vi "Main.vi"(11 "Module Admin":refnum<class "Delacor_lib_QMH_Cloneable Module Admin.lvclass">) -> ()   [LabVIEW 2024, in "CTIWrapper.lvlib"]
doc: "This template is based off of the Queued Message Handler design pattern and the Queued Message Handler project template that ships with LabVIEW.\n\nThe main difference is that the queue is private to this module and communication between modules is performed via Broadcast and Request events.\n\nRequest events are wrapped in public API methods and are handled in the Event Handling Loop (EHL) of this VI. Any module can register for Broadcast events sent by this module. The EHL generates messages based on user interface actions.\n\nThe Message Handling Loop (MHL) processes messages generated by the EHL, or by other messages. The messages are string values, so new messages can be added easily to the Message Cases case structure in the MHL. Each message cluster can also provide an optional value for Message Data, which is a variant that can be converted to whatever message-specific data is required.\n_____\nBased on DQMH Dev Tools: Project Template 7.1.0.1503."
uses:
  CTIWrapper.lvlib
  <vilib>/Delacor/Delacor QMH/Libraries/Cloneable Module Admin_class/Delacor_lib_QMH_Cloneable Module Admin.lvclass
  C:/Program Files (x86)/National Instruments/LabVIEW 2024/vi.lib/Delacor/Delacor QMH/Libraries/Module Admin_class/Delacor_lib_QMH_Module Admin.lvclass
  Module Data--cluster.ctl
  <vilib>/Delacor/Delacor QMH/Libraries/Cloneable Module Admin_class/Delacor_lib_QMH_Cloneable Module Admin.lvclass/Delacor_lib_QMH_Cloneable Module Admin.ctl
  <vilib>/Delacor/Delacor QMH/Libraries/Message Queue_class/Delacor_lib_QMH_Message Queue.lvclass/Delacor_lib_QMH_Message Queue.ctl
  Stop Argument--cluster.ctl
  <vilib>/Delacor/Delacor QMH/Libraries/Module Admin_class/Delacor_lib_QMH_Module Admin.lvclass/Delacor_lib_QMH_Module Admin.ctl
  Initialize Device Argument--cluster.ctl
  Initialize Device (Reply Payload)--cluster.ctl
  <instrlib>/HandsOnPi2040/cti-drivers-lv-visa-main/CTI-Visa/Identity.ctl
  Set DO Argument--cluster.ctl
  Close Device Argument--cluster.ctl
  <vilib>/Utility/miscctls.llb/LVPointTypeDef.ctl
  <vilib>/Delacor/Delacor QMH/Libraries/Message Queue_class/Delacor_lib_QMH_Enqueue Message (Single).vi
  <vilib>/Delacor/Delacor QMH/Libraries/Cloneable Module Admin_class/Delacor_lib_QMH_Get Module ID.vi
  <vilib>/Delacor/Delacor QMH/Libraries/Module Admin_class/Delacor_lib_QMH_Get External Launch.vi
  <vilib>/Delacor/Delacor QMH/Libraries/Message Queue_class/Delacor_lib_QMH_Message Queue.lvclass
  <instrlib>/HandsOnPi2040/cti-drivers-lv-visa-main/CTI-Visa/CTI-Visa.lvlib
  <instrlib>/HandsOnPi2040/HandsOnPi2040.lvlib
panel:
  out "Digital Inputs":bool[](array[boolean])
  out "Connection Status":bool
  in  "VISA resource name":refnum<visa-resource-name>
  in  "Initialize Device":bool
  out "error out":errorcluster
  out "Status":string
  in  "Simulate EHL Error":bool
  in  "Simulate MHL Error":bool
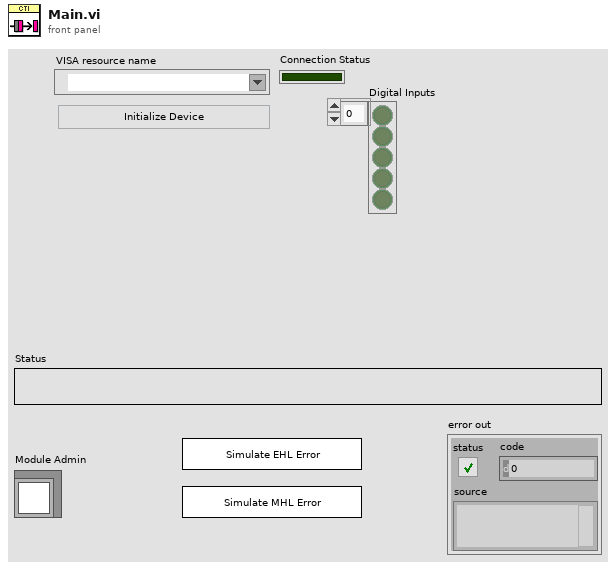
[diagram p1: front panel]
types:
  T1 = typedef "CTIWrapper.lvlib/Request Events--cluster.ctl" = cluster{"Stop Module":refnum<user-event>, "Show Panel":refnum<user-event>, "Hide Panel":refnum<user-event>, "Show Diagram":refnum<user-event>, "Get Module Execution Status":refnum<user-event>, "Initialize Device":refnum<user-event>, "Local Instance":T2, "Set DO":refnum<user-event>, "Close Device":refnum<user-event>}
  T2 = typedef "CTIWrapper.lvlib/Local Instance Request Events--cluster.ctl" = cluster{"Wake Up CT HL":refnum<user-event>}
  T3 = typedef "CTIWrapper.lvlib/Module Data--cluster.ctl" = cluster{"Status":string, "VISA resource name":refnum<visa-resource-name>, "Connected?":bool}
  T4 = enum32{"invalid lock state", "Not Locked", "Locked (No Password)", "Password-protected"}
  T5 = typedef "CTIWrapper.lvlib/Stop Argument--cluster.ctl" = cluster{"Module ID":i32, "Origin":string, "Exit via Stop Module Req?":bool, "Wait for Module to stop?":bool}
  T6 = typedef "CTIWrapper.lvlib/Initialize Device Argument--cluster.ctl" = cluster{"Module ID":i32, "VISA resource name":refnum<visa-resource-name>, "Wait Notifier":refnum<notifier>, "wait for reply":bool}
  T7 = typedef "CTIWrapper.lvlib/Set DO Argument--cluster.ctl" = cluster{"Module ID":i32, "Digital Outputs":bool[]}
  T8 = typedef "CTIWrapper.lvlib/Close Device Argument--cluster.ctl" = cluster{"Module ID":i32, "Boolean":bool}
  T9 = typedef "LVPointTypeDef.ctl" = cluster{"Horizontal":i16, "Vertical":i16}
  T10 = enum32{"Invalid", "Standard", "Closed", "Hidden", "Minimized", "Maximized"}
  T11 = typedef "CTIWrapper.lvlib/Initialize Device (Reply Payload)--cluster.ctl" = cluster{"Module ID":i32, "Identity":T12, "error":errorcluster}
  T12 = typedef "CTI-Visa.lvlib/Identity.ctl" = cluster{"Vendor":string, "Model":string, "Serial":string, "Version":string}
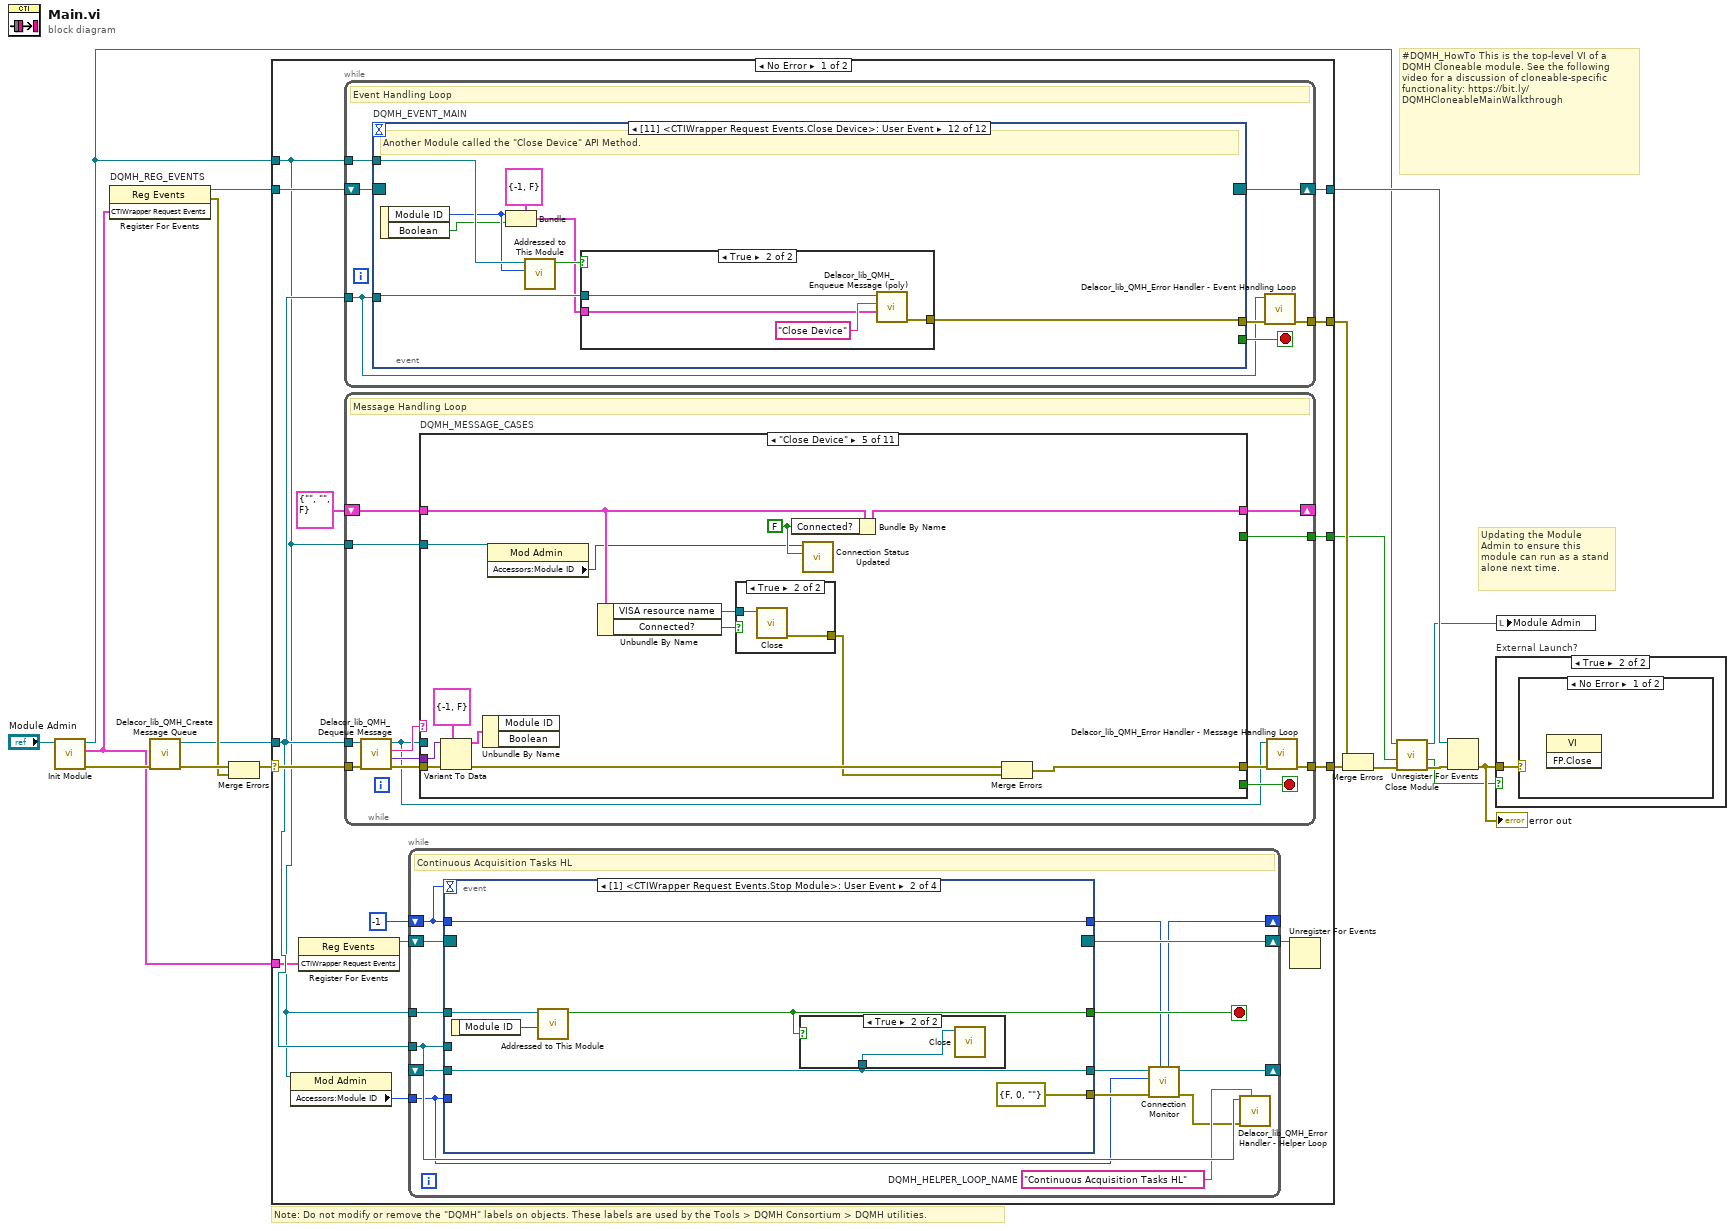
[diagram p0: block diagram]
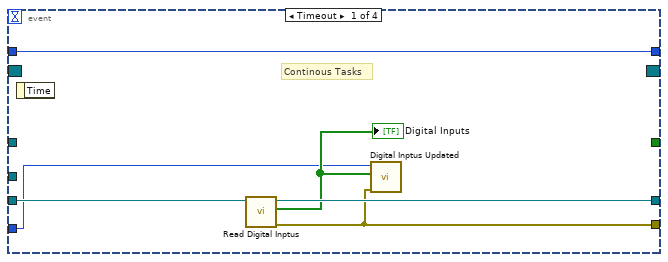
[diagram p2: hidden frame]
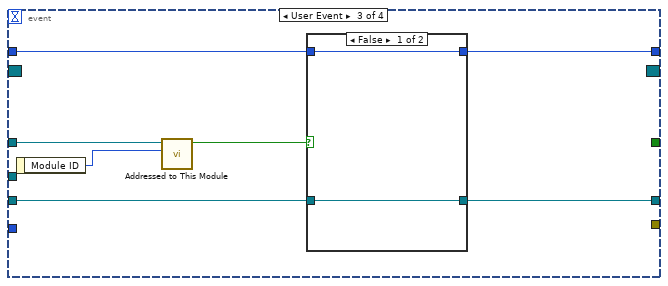
[diagram p4: hidden frame]
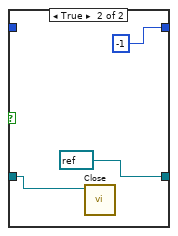
[diagram p5: hidden frame]
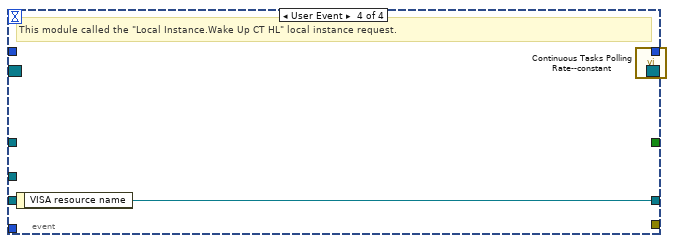
[diagram p6: hidden frame]
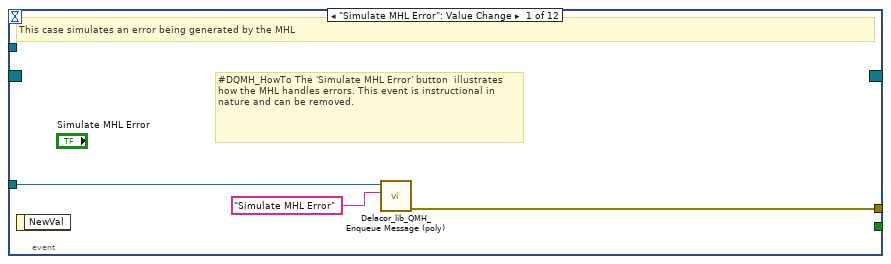
[diagram p7: hidden frame]
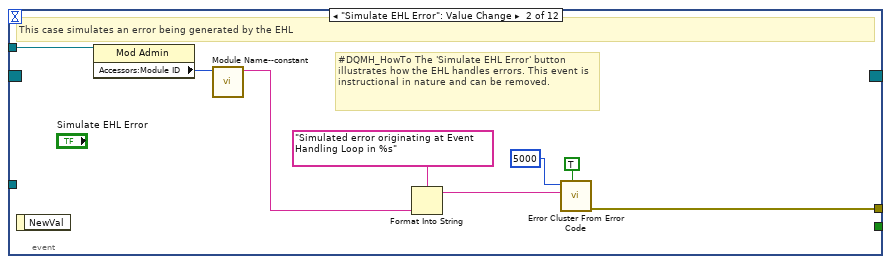
[diagram p8: hidden frame]
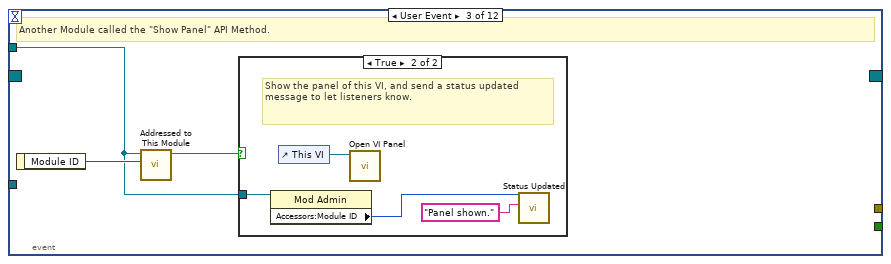
[diagram p9: hidden frame]
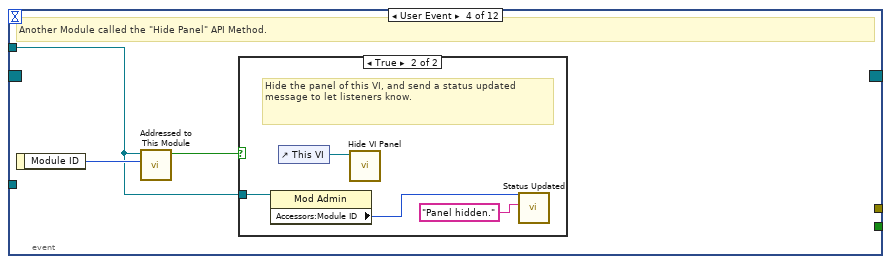
[diagram p11: hidden frame]
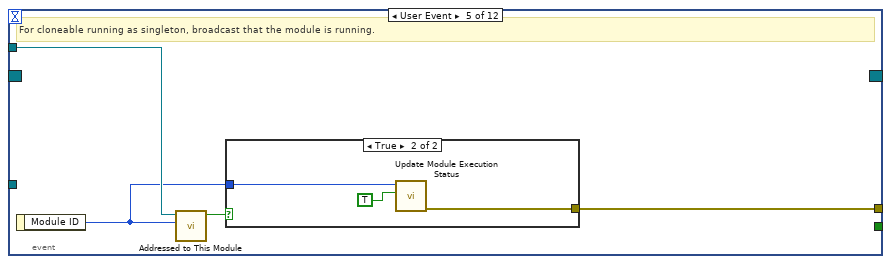
[diagram p13: hidden frame]
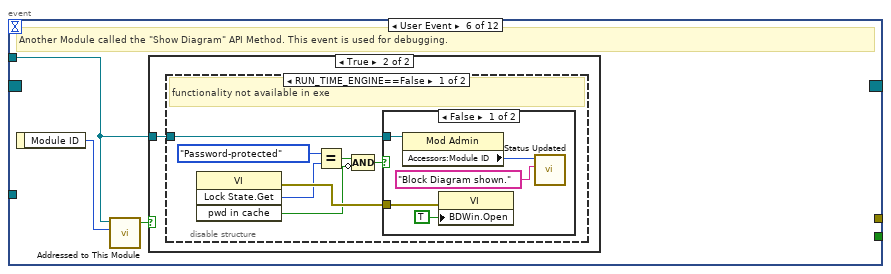
[diagram p15: hidden frame]
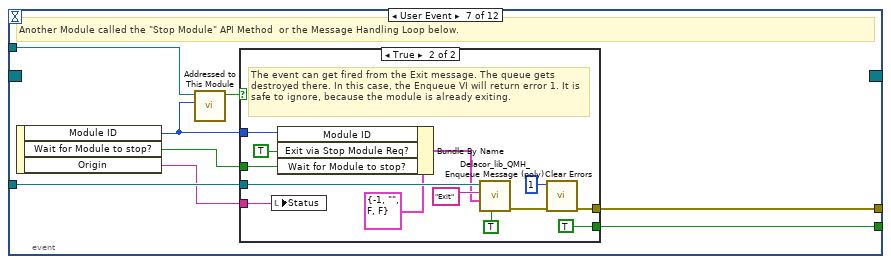
[diagram p19: hidden frame]
diagram:
  # "#DQMH_HowTo This is the top-level VI of a DQMH Cloneable module. See the following video for a discussion of cloneable-specific functionality: https://bit.ly/DQMHCloneableMainWalkthrough"
  # "Note: Do not modify or remove the \"DQMH\" labels on objects. These labels are used by the Tools > DQMH Consortium > DQMH utilities."
  # "Updating the Module Admin to ensure this module can run as a stand alone next time."
  n1 = call "Init Module.vi"("Cloneable Module Admin in"="Module Admin") -> ("error out"=w15:errorcluster, "CTIWrapper Request Events"=w1:T1, "Cloneable Module Admin out"=w5:refnum<class "Delacor_lib_QMH_Cloneable Module Admin.lvclass">)  [unwired: 8 in]
  n2 = register-events "DQMH_REG_EVENTS"(w1) -> (reference out=w8:refnum<event-registration>, error out=w10:errorcluster)  [unwired: 2 in]
  n3 = call <vilib>:"Delacor_lib_QMH_Create Message Queue.vi"("error in"=w15) -> ("error out"=w12:errorcluster, "Message Queue"=w7:refnum<class "Delacor_lib_QMH_Message Queue.lvclass">)  [unwired: 9 in]
  n4 = Merge Errors(w12, w10) -> (w11:errorcluster)
  n5 = case shown="No Error" w11 {
    selector: w11 -> [w30 w379]
    tunnel: [w32 w378] -> w16
    tunnel: [w29 w377] -> w9
    tunnel: w8 -> [w27 w377]
    tunnel: w7 -> [w26 w370]
    tunnel: [w31 _] -> w17
    tunnel: w5 -> [w20 w373]
    tunnel: [w25 _] -> w3
    tunnel: w1 -> [w24 _]
    frame No Error {
      n6 = property class="Mod Admin"(reference=w20) -> ("Accessors:Module ID"=w19:i32)  [unwired: 1 in, 2 out]
      n7 = register-events ("DQMH_HELPER_REGFOREVENTS")(w24) -> (reference out=w22:refnum<event-registration>)  [unwired: 2 in, 1 out]
      n8 = while {
        tunnel: w26 -> [w75]
        shift-right: [w78] -> w29
        shift-left: w27 -> [w79]
        tunnel: [w80] -> w31
        tunnel: w20 -> [w76]
        stop <- w77 stop-if-true
        # "Event Handling Loop"
        n9 = event "DQMH_EVENT_MAIN" shown="[11] <CTIWrapper Request Events.Close Device>: User Event" {
          selector: w79 -> [_ _ _ _ _ _ _ _ _ _ _ _]
          dyn-events: [_ _ _ _ _ _ _ _ _ _ _ _] -> w78
          timeout: _ -> [_ _ _ _ _ _ _ _ _ _ _ _]
          tunnel: [_ _ _ _ _ _ w133 _ _ _ _ _] -> w77
          tunnel: w75 -> [w83 _ _ _ _ _ w136 w153 w175 w186 w194 w206]
          tunnel: [w84 w92 _ _ w110 _ w137 w156 w166 w183 w187 w199] -> w81
          tunnel: w76 -> [_ w91 w93 w100 w108 w114 w135 w154 w173 _ w192 w204]
          event "Simulate MHL Error": Value Change {
            # "#DQMH_HowTo The 'Simulate MHL Error' button  illustrates how the MHL handles errors. This event is instructional in nature and can be removed."
            # "This case simulates an error being generated by the MHL"
            n10 = event-data() -> ()  [unwired: 1 in, 1 out]
            n11 = call-poly <vilib>:"Delacor_lib_QMH_Enqueue Message (poly).vi"("Message"="Simulate MHL Error", "Message Queue in"=w83) -> ("error out"=w84:errorcluster)  [unwired: 8 in, 1 out]
          }
          event "Simulate EHL Error": Value Change {
            # "#DQMH_HowTo The 'Simulate EHL Error' button  illustrates how the EHL handles errors. This event is instructional in nature and can be removed."
            # "This case simulates an error being generated by the EHL"
            n12 = event-data() -> ()  [unwired: 1 in, 1 out]
            n13 = property on="Property Node" class="Mod Admin"(reference=w91) -> ("Accessors:Module ID"=w90:i32)  [unwired: 1 in, 2 out]
            n14 = call "Module Name--constant.vi"("Module ID"=w90) -> ("Module Name"=w85:string)  [unwired: 10 in]
            n15 = Format Into String(format string="Simulated error originating at Event Handling Loop in %s", w85) -> (resulting string=w88:string)  [unwired: 2 in, 1 out]
            n16 = call <vilib>:"Error Cluster From Error Code.vi"("show call chain? (False)"=TRUE, "error message (\"\")"=w88, "error code (0)"=5000) -> ("error out"=w92:errorcluster)  [unwired: 6 in]
          }
          event User Event {
            # "Another Module called the \"Show Panel\" API Method."
            n17 = event-data() -> ("Module ID"=w94:i32)  [unwired: 1 in]
            n18 = call "Addressed to This Module.vi"("Module ID from Argument"=w94, "Module Admin"=w93) -> ("Addressed to this instance?"=w95:bool)  [unwired: 8 in, 1 out]
            n19 = case shown="True" w95 {
              tunnel: w93 -> [_ w97]
              frame False {
              }
              frame True {
                # "Show the panel of this VI, and send a status updated message to let listeners know."
                n20 = property on="Property Node" class="Mod Admin"(reference=w97) -> ("Accessors:Module ID"=w96:i32)  [unwired: 1 in, 2 out]
                n21 = control-ref of="This VI"() -> (w99:refnum<vi>)
                n22 = call "Open VI Panel.vi"("VI"=w99) -> ()  [unwired: 10 in, 1 out]
                n23 = call "Status Updated.vi"("Status"="Panel shown." ("format string"), "Module ID"=w96) -> ()  [unwired: 9 in, 1 out]
              }
            }
          }
          event User Event {
            # "Another Module called the \"Hide Panel\" API Method."
            n24 = event-data() -> ("Module ID"=w101:i32)  [unwired: 1 in]
            n25 = call "Addressed to This Module.vi"("Module ID from Argument"=w101, "Module Admin"=w100) -> ("Addressed to this instance?"=w102:bool)  [unwired: 8 in, 1 out]
            n26 = case shown="True" w102 {
              tunnel: w100 -> [_ w104]
              frame False {
              }
              frame True {
                # "Hide the panel of this VI, and send a status updated message to let listeners know."
                n27 = property on="Property Node" class="Mod Admin"(reference=w104) -> ("Accessors:Module ID"=w103:i32)  [unwired: 1 in, 2 out]
                n28 = control-ref of="This VI"() -> (w106:refnum<vi>)
                n29 = call "Hide VI Panel.vi"("VI"=w106) -> ()  [unwired: 10 in, 1 out]
                n30 = call "Status Updated.vi"("Status"="Panel hidden." ("format string"), "Module ID"=w103) -> ()  [unwired: 9 in, 1 out]
              }
            }
          }
          event User Event {
            # "For cloneable running as singleton, broadcast that the module is running."
            n31 = event-data() -> ("Module ID"=w107:i32)  [unwired: 1 in]
            n32 = call "Addressed to This Module.vi"("Module ID from Argument"=w107, "Module Admin"=w108) -> ("Addressed to this instance?"=w109:bool)  [unwired: 8 in, 1 out]
            n33 = case shown="True" w109 {
              tunnel: [_ w113] -> w110
              tunnel: w107 -> [_ w112]
              frame False {
              }
              frame True {
                n34 = call "Update Module Execution Status.vi"("Running?"=TRUE, "Module ID"=w112) -> ("error out"=w113:errorcluster)  [unwired: 9 in]
              }
            }
          }
          event User Event {
            # "Another Module called the \"Show Diagram\" API Method. This event is used for debugging."
            n35 = event-data() -> ("Module ID"=w115:i32)  [unwired: 1 in]
            n36 = call "Addressed to This Module.vi"("Module ID from Argument"=w115, "Module Admin"=w114) -> ("Addressed to this instance?"=w116:bool)  [unwired: 8 in, 1 out]
            n37 = case shown="True" w116 {
              tunnel: w114 -> [_ w117]
              frame False {
              }
              frame True {
                n38 = disable-structure shown="RUN_TIME_ENGINE==False" {
                  disable-tunnel: w117 -> [w118 _]
                  frame condition #0 (active) {
                    # "functionality not available in exe"
                    n39 = invoke on="Invoke Node" class="VI" method="Lock State.Get"() -> (error out=w124:errorcluster, "Get Lock State"=w123:T4, "pwd in cache"=w120:bool)  [unwired: 4 in, 1 out]
                    n40 = Equal?(x=T4."Password-protected", y=w123) -> (x = y?=w121:bool)
                    n41 = Compound Arithmetic op=AND(w121, invert w120) -> (w119:bool)
                    n42 = case shown="False" w119 {
                      tunnel: w124 -> [w129 _]
                      tunnel: w118 -> [w126 _]
                      frame False {
                        n43 = property on="Property Node" class="Mod Admin"(reference=w126) -> ("Accessors:Module ID"=w125:i32)  [unwired: 1 in, 2 out]
                        n44 = property on="Property Node" class="VI"(error in=w129, "BDWin.Open"=TRUE ("Block Diagram Window:Open")) -> ()  [unwired: 1 in, 2 out]
                        n45 = call "Status Updated.vi"("Status"="Block Diagram shown." ("format string"), "Module ID"=w125) -> ()  [unwired: 9 in, 1 out]
                      }
                      frame True {
                        # "Password-protected VI, and the password is not in the cache. Do not show the diagram."
                      }
                    }
                  }
                  frame condition #1 {
                  }
                }
              }
            }
          }
          event User Event {
            # "Another Module called the \"Stop Module\" API Method  or the Message Handling Loop below."
            n46 = event-data() -> ("Module ID"=w131:i32, "Wait for Module to stop?"=w132:bool, "Origin"=w130:string)  [unwired: 1 in]
            n47 = call "Addressed to This Module.vi"("Module ID from Argument"=w131, "Module Admin"=w135) -> ("Addressed to this instance?"=w134:bool)  [unwired: 8 in, 1 out]
            n48 = case shown="True" w134 {
              tunnel: [_ w149] -> w137
              tunnel: w136 -> [_ w145]
              tunnel: [_ TRUE] -> w133
              tunnel: w132 -> [_ w140]
              tunnel: w131 -> [_ w142]
              tunnel: w130 -> [_ w138]
              frame False {
              }
              frame True {
                # "The event can get fired from the Exit message. The queue gets destroyed there. In this case, the Enqueue VI will return error 1. It is safe to ignore, because the module is already exiting."
                n49 = local write "Status"(w138) -> ()
                n50 = Bundle By Name(cluster=T5 {"Module ID"=-1, "Origin"="", "Exit via Stop Module Req?"=FALSE, "Wait for Module to stop?"=FALSE} ("Stop Argument"), "Module ID"=w142, "Exit via Stop Module Req?"=TRUE, "Wait for Module to stop?"=w140) -> (w139:T5)
                n51 = call-poly <vilib>:"Delacor_lib_QMH_Enqueue Message (poly).vi"("Priority Message? (F)"=TRUE, "Message Data"=w139, "Message"="Exit", "Message Queue in"=w145) -> ("error out"=w150:errorcluster)  [unwired: 6 in, 1 out]
                n52 = call <vilib>:"Clear Errors.vi"("error in (no error)"=w150, "specific error code to clear (0: all)"=1) -> ("error out"=w149:errorcluster)  [unwired: 4 in, 1 out]
              }
            }
          }
          event Panel Close? {
            w155 = TRUE  # Discard the event, the MHL is responsible for closing and stopping this VI.
            # "Hide the panel or send the 'Exit' message if the user clicks the 'X' on the module main VI panel."
            n53 = event-data() -> ()  [unwired: 1 in, 1 out]
            n54 = property on="Property Node" class="Mod Admin"(reference=w154) -> (reference out=w151:refnum<class "Delacor_lib_QMH_Cloneable Module Admin.lvclass">, "Accessors:External Launch"=w152:bool)  [unwired: 1 in, 1 out]
            n55 = case shown="True" w152 {
              tunnel: w153 -> [_ w164]
              tunnel: [_ w165] -> w156
              tunnel: w151 -> [w159 _]
              frame True {
                # "If externally launched, clicking the 'X' hides the panel, but doesn't close it."
                n56 = property on="Property Node" class="Mod Admin"(reference=w159) -> ("Accessors:Module ID"=w158:i32)  [unwired: 1 in, 2 out]
                n57 = call "Status Updated.vi"("Status"="Panel hidden." ("format string"), "Module ID"=w158) -> ("error out"=w157:errorcluster)  [unwired: 9 in]
                n58 = control-ref of="This VI"() -> (w161:refnum<vi>)
                n59 = call "Hide VI Panel.vi"("error in"=w157, "VI"=w161) -> ()  [unwired: 9 in, 1 out]
              }
              frame False {
                # "If run as a stand-alone VI, clicking the panel 'X' stops the VI."
                n60 = call-poly <vilib>:"Delacor_lib_QMH_Enqueue Message (poly).vi"("Priority Message? (F)"=TRUE, "Message"="Exit", "Message Queue in"=w164) -> ("error out"=w165:errorcluster)  [unwired: 7 in, 1 out]
              }
            }
            n61 = event-data ("Event Filter Node")("Discard?"=w155) -> ()  [unwired: 1 in, 1 out]
          }
          event User Event {
            # "Another Module called the \"Initialize Device\" API Method."
            n62 = event-data() -> ("Module ID"=w170:i32, "VISA resource name"=w169:refnum<visa-resource-name>, "Wait Notifier"=w168:refnum<notifier>, "wait for reply"=w167:bool)  [unwired: 1 in]
            n63 = Bundle(cluster=T6 {"Module ID"=-1, "VISA resource name"="", "Wait Notifier"=refnum, "wait for reply"=FALSE} ("Initialize Device Argument"), "Module ID"=w170, "VISA resource name"=w169, "Wait Notifier"=w168, "wait for reply"=w167) -> (w171:T6)
            n64 = call "Addressed to This Module.vi"("Module ID from Argument"=w170, "Module Admin"=w173) -> ("Addressed to this instance?"=w174:bool)  [unwired: 8 in, 1 out]
            n65 = case shown="True" w174 {
              tunnel: w175 -> [_ w179]
              tunnel: w171 -> [_ w177]
              tunnel: [_ w176] -> w166
              frame False {
              }
              frame True {
                n66 = call-poly <vilib>:"Delacor_lib_QMH_Enqueue Message (poly).vi"("Message Data"=w177, "Message"="Initialize Device", "Message Queue in"=w179) -> ("error out"=w176:errorcluster)  [unwired: 7 in, 1 out]
              }
            }
          }
          event "Initialize Device": Value Change {
            # "Another Module called the \"Initialize Device\" API Method."
            n67 = event-data() -> ()  [unwired: 1 in, 1 out]
            n68 = Bundle(cluster=T6 {"Module ID"=-1, "VISA resource name"="", "Wait Notifier"=refnum, "wait for reply"=FALSE} ("Initialize Device Argument"), "VISA resource name"="VISA resource name", "wait for reply"=FALSE) -> (w184:T6)  [unwired: 2 in]
            n69 = call-poly <vilib>:"Delacor_lib_QMH_Enqueue Message (poly).vi"("Message Data"=w184, "Message"="Initialize Device", "Message Queue in"=w186) -> ("error out"=w183:errorcluster)  [unwired: 7 in, 1 out]
          }
          event User Event {
            # "Another Module called the \"Set DO\" API Method."
            n70 = event-data() -> ("Module ID"=w189:i32, "Digital Outputs"=w188:bool[])  [unwired: 1 in]
            n71 = Bundle(cluster=T7 {"Module ID"=-1, "Digital Outputs"=[]} ("Set DO Argument"), "Module ID"=w189, "Digital Outputs"=w188) -> (w190:T7)
            n72 = call "Addressed to This Module.vi"("Module ID from Argument"=w189, "Module Admin"=w192) -> ("Addressed to this instance?"=w193:bool)  [unwired: 8 in, 1 out]
            n73 = case shown="True" w193 {
              tunnel: w194 -> [_ w198]
              tunnel: w190 -> [_ w196]
              tunnel: [_ w195] -> w187
              frame False {
              }
              frame True {
                n74 = call-poly <vilib>:"Delacor_lib_QMH_Enqueue Message (poly).vi"("Message Data"=w196, "Message"="Set DO", "Message Queue in"=w198) -> ("error out"=w195:errorcluster)  [unwired: 7 in, 1 out]
              }
            }
          }
          event User Event {
            # "Another Module called the \"Close Device\" API Method."
            n75 = event-data() -> ("Module ID"=w201:i32, "Boolean"=w200:bool)  [unwired: 1 in]
            n76 = Bundle(cluster=T8 {"Module ID"=-1, "Boolean"=FALSE} ("Close Device Argument"), "Module ID"=w201, "Boolean"=w200) -> (w202:T8)
            n77 = call "Addressed to This Module.vi"("Module ID from Argument"=w201, "Module Admin"=w204) -> ("Addressed to this instance?"=w205:bool)  [unwired: 8 in, 1 out]
            n78 = case shown="True" w205 {
              tunnel: w206 -> [_ w210]
              tunnel: w202 -> [_ w208]
              tunnel: [_ w207] -> w199
              frame False {
              }
              frame True {
                n79 = call-poly <vilib>:"Delacor_lib_QMH_Enqueue Message (poly).vi"("Message Data"=w208, "Message"="Close Device", "Message Queue in"=w210) -> ("error out"=w207:errorcluster)  [unwired: 7 in, 1 out]
              }
            }
          }
        }
        n80 = call-dynamic "Delacor_lib_QMH_Error Handler - Event Handling Loop.vi"("error in"=w81, "Message Queue in"=w75) -> ("dup error in"=w80:errorcluster)  [unwired: 8 in, 1 out]
      }
      n81 = while {
        tunnel: w26 -> [w211]
        shift-right: [w218] -> _
        shift-left: T3 {"Status"="", "VISA resource name"="", "Connected?"=FALSE} ("Data Cluster") -> [w219]
        tunnel: w30 -> [w222]
        tunnel: [w220] -> w32
        tunnel: w20 -> [w213]
        tunnel: [w212] -> w25
        stop <- w217 stop-if-true
        # "Message Handling Loop"
        n82 = call-dynamic "Delacor_lib_QMH_Dequeue Message.vi"("error in"=w222, "Message Queue in"=w211) -> ("error out"=w221:errorcluster, "Message Data"=w215:variant, "Message"=w216:string, "Message Queue out"=w214:refnum<class "Delacor_lib_QMH_Message Queue.lvclass">)  [unwired: 6 in]
        n83 = case "DQMH_MESSAGE_CASES" shown="\"Close Device\"" w216 {
          selector: w216 -> [_ _ _ _ _ _ _ _ _ _ w359]
          tunnel: w214 -> [_ _ _ _ _ _ _ w313 _ w351 _]
          tunnel: w221 -> [w242 w246 w265 w280 w303 w308 w310 w322 w339 w357 w368]
          tunnel: [w240 w246 w255 w272 w294 w307 w310 w318 w338 w352 w369] -> w223
          tunnel: w219 -> [w233 w245 w264 w274 w297 w306 w309 w317 w336 w341 w366]
          tunnel: [w232 w245 w250 w274 w298 w306 w309 w317 w336 w341 w366] -> w218
          tunnel: [_ _ _ _ _ _ _ _ _ w350 _] -> w217
          tunnel: w215 -> [_ _ w262 w278 w301 _ _ w316 _ w348 _]
          tunnel: w213 -> [w228 _ w254 w269 w291 _ _ w315 w334 w343 w365]
          tunnel: [_ _ _ _ _ _ _ _ _ w346 _] -> w212
          frame "Initialize" {
            w225 = "Initial Message" ("Initial Message")
            # "#DQMH_CodeNeeded - Initialize the appearance of the front panel."
            # "#DQMH_CodeNeeded - Initialize your state data here."
            # "Initialize - Any operation that needs to be done before the module can receive messages. Synchronize Caller Events.vi will inform Start Module.vi that the module has launched and is ready to receive messages. Module Did Init.vi will broadcast that the module initialized."
            n84 = call "Synchronize Caller Events.vi"("error in"=w242, "Module Admin"=w228) -> ("error out"=w241:errorcluster, "Module Admin out"=w227:refnum<class "Delacor_lib_QMH_Cloneable Module Admin.lvclass">)  [unwired: 8 in]
            n85 = property on="Property Node" class="Mod Admin"(reference=w227) -> ("Accessors:Module ID"=w224:i32, "Accessors:External Launch"=w229:bool)  [unwired: 1 in, 2 out]
            n86 = call "Module Name--constant.vi"("Module ID"=w224) -> ("Module Name"=w237:string)  [unwired: 10 in]
            n87 = property on="Property Node" class="VI"("Front Panel.Title"=w237) -> (reference out=w239:refnum<vi>, error out=w244:errorcluster)  [unwired: 2 in]
            n88 = Select(t=T10."Hidden" ("State"), s=w229, f=T10."Standard" ("State")) -> (s? t:f=w234:T10)
            n89 = invoke on="Invoke Node" class="VI" method="FP.Open"(reference=w239, error in=w244, "State"=w234) -> (reference out=w238:refnum<vi>, error out=w243:errorcluster)  [unwired: 2 in, 3 out]
            n90 = Bundle By Name(cluster=w233, "Status"=w225) -> (w232:T3)
            n91 = invoke on="Invoke Node" class="VI" method="FP.Center"(reference=w238, error in=w243) -> ()  [unwired: 1 in, 3 out]
            n92 = property on="Pane" class="Pane"("Origin"=T9 {"Horizontal"=0, "Vertical"=0}) -> ()  [unwired: 2 in, 2 out]
            n93 = call "Module Name--constant.vi"("Module ID"=w224) -> ("Module Name"=w230:string)  [unwired: 10 in]
            n94 = call "Module Did Init.vi"("error in"=w241, "Initialized?"=TRUE, "Origin"=w230, "Module ID"=w224) -> ("error out"=w240:errorcluster)  [unwired: 7 in]
            "Status" <- w225
          }
          frame "---Module Specific---" {
            # "Separator -- The following cases handle messages specific to this Module."
          }
          frame "Initialize Device" {
            # "Initialize Device"
            n95 = property class="Mod Admin"(reference=w254) -> ("Accessors:Module ID"=w251:i32)  [unwired: 1 in, 2 out]
            n96 = Variant To Data(error in=w265, type=T6 {"Module ID"=-1, "VISA resource name"="", "Wait Notifier"=refnum, "wait for reply"=FALSE} ("Initialize Device Argument"), Variant=w262) -> (data=w260:T6, error out=w263:errorcluster)
            n97 = Unbundle By Name(w260) -> ("VISA resource name"=w253:refnum<visa-resource-name>, "Wait Notifier"=w259:refnum<notifier>, "wait for reply"=w258:bool)  [unwired: 1 out]
            n98 = call <instrlib>:"Initialize.vi"("VISA resource name"=w253) -> ("error out"=w247:errorcluster, "Identity"=w252:T12, "VISA resource name out"=w249:refnum<visa-resource-name>)  [unwired: 8 in]
            n99 = Not(x=w247) -> (.not. x?=w248:bool)
            "Connection Status" <- w248
            n100 = Bundle By Name(cluster=w264, "VISA resource name"=w249, "Connected?"=w248) -> (w250:T3)
            n101 = call "Connection Status Updated.vi"("error in"=w247, "Connected?"=w248, "Module ID"=w251) -> ()  [unwired: 8 in, 1 out]
            n102 = Bundle By Name(cluster=T11 {"Module ID"=-1, "Identity"={"Vendor"="", "Model"="", "Serial"="", "Version"=""}, "error"={"status"=FALSE, "code"=0, "source"=""}} ("Initialize Device (Reply Payload)"), "Module ID"=w251, "Identity"=w252, "error"=w247) -> (w257:T11)
            n103 = Merge Errors(w263, w247) -> (w255:errorcluster)
            n104 = call "Wake Up CT HL.vi"("error in"=w247, "VISA resource name"=w249, "Module ID"=w251) -> ()  [unwired: 8 in, 1 out]
            n105 = case "DQMH_FIRE_NOTIFIER" shown="False" w258 {
              tunnel: w259 -> [_ w267]
              tunnel: w257 -> [_ w266]
              frame False {
              }
              frame True {
                n106 = Send Notification(notification=w266, notifier=w267) -> ()  [unwired: 1 in, 2 out]
              }
            }
          }
          frame "Set DO" {
            n107 = Variant To Data(error in=w280, type=T7 {"Module ID"=-1, "Digital Outputs"=[]} ("Set DO Argument"), Variant=w278) -> (data=w276:T7, error out=w279:errorcluster)
            n108 = property class="Mod Admin"(reference=w269) -> ("Accessors:Module ID"=w268:i32)  [unwired: 1 in, 2 out]
            n109 = Unbundle By Name(w276) -> ("Digital Outputs"=w275:bool[])  [unwired: 1 out]
            n110 = Unbundle By Name(w274) -> ("VISA resource name"=w273:refnum<visa-resource-name>, "Connected?"=w270:bool)
            n111 = case shown="True" w270 {
              tunnel: w275 -> [_ w287]
              tunnel: w273 -> [w282 w286]
              tunnel: [w283 w284] -> w271
              tunnel: w268 -> [w281 w285]
              frame False {
                n112 = call "CTI Device Not Connected--error.vi"("Module ID"=w281, "VISA resource name"=w282) -> ("error out"=w283:errorcluster)  [unwired: 9 in]
              }
              frame True {
                n113 = call "Write Digital Outputs.vi"("Digital Outputs"=w287, "VISA Refnum in"=w286) -> ("error out"=w284:errorcluster)  [unwired: 8 in, 1 out]
                n114 = case shown="Error .." w284 {
                  selector: w284 -> [_ w288]
                  tunnel: w285 -> [_ w289]
                  frame No Error {
                  }
                  frame Error {
                    n115 = call "Close Device.vi"("error in"=w288, "Module ID"=w289) -> ()  [unwired: 9 in, 1 out]
                  }
                }
              }
            }
            n116 = Merge Errors(w279, w271) -> (w272:errorcluster)
          }
          frame "Close Device" {
            w292 = FALSE ("Connected?")
            n117 = Variant To Data(error in=w303, type=T8 {"Module ID"=-1, "Boolean"=FALSE} ("Close Device Argument"), Variant=w301) -> (data=w299:T8, error out=w302:errorcluster)
            n118 = Unbundle By Name(w299) -> ()  [unwired: 2 out]
            n119 = property class="Mod Admin"(reference=w291) -> ("Accessors:Module ID"=w290:i32)  [unwired: 1 in, 2 out]
            n120 = Unbundle By Name(w297) -> ("VISA resource name"=w296:refnum<visa-resource-name>, "Connected?"=w295:bool)
            n121 = case shown="True" w295 {
              tunnel: w296 -> [_ w305]
              tunnel: [_ w304] -> w293
              frame False {
              }
              frame True {
                n122 = call <instrlib>:"Close.vi"("VISA resource name"=w305) -> ("error out"=w304:errorcluster)  [unwired: 10 in]
              }
            }
            n123 = Bundle By Name(cluster=w297, "Connected?"=w292) -> (w298:T3)
            n124 = call "Connection Status Updated.vi"("Connected?"=w292, "Module ID"=w290) -> ()  [unwired: 9 in, 1 out]
            n125 = Merge Errors(w302, w293) -> (w294:errorcluster)
          }
          frame "---Copy This Frame---" {
            # "Duplicate this frame when creating new messages.  Change this comment in the duplicated frame to describe this message."
            n126 = Merge Errors(w308) -> (w307:errorcluster)
          }
          frame "---Exit and Error Handling---" {
            # "Separator - the following cases handle errors and exit messages."
          }
          frame "Error" {
            # "#DQMH_CodeRecommended - If the module is running in standalone mode (External Launch = FALSE), this code will pop up an error dialog and call the 'Exit' message if an error occurs. Add more fine-grained error management here."
            # "Error - Check the error message data and respond accordingly. This message is sent by the \"Error Handler\" VIs at the end of each loop in this application."
            n127 = property on="Property Node" class="Mod Admin"(reference=w315) -> ("Accessors:External Launch"=w314:bool, "Accessors:Module ID"=w312:i32)  [unwired: 1 in, 2 out]
            n128 = Variant To Data(error in=w322, type=errorcluster {"status"=FALSE, "code"=0, "source"=""} ("error constant"), Variant=w316) -> (data=w311:errorcluster, error out=w320:errorcluster)
            n129 = local write "error out"(w311) -> ()
            n130 = call "Error Reported.vi"("Error"=w311, "Module ID"=w312) -> ()  [unwired: 9 in, 1 out]
            n131 = case shown="False" w314 {
              tunnel: [w327 _] -> w319
              tunnel: w313 -> [w325 _]
              tunnel: w311 -> [w326 _]
              frame False {
                n132 = disable-structure shown="Default" {
                  disable-tunnel: w326 -> [w328 _]
                  frame condition #0 (active) {
                    # "If the module is running standalone, then pop up an error dialog and call the \"Exit\" message."
                    n133 = call <vilib>:"Simple Error Handler.vi"("error in (no error)"=w328) -> ()  [unwired: 4 in, 5 out]
                  }
                  frame condition #1 {
                    # "To prevent the Simple Error Handler VI from being loaded (e.g. when deploying to a Real-Time target), add the Conditional Disable Symbol \"DQMH_Disable_SEH\" to your project and set it to TRUE."
                  }
                }
                n134 = call-poly <vilib>:"Delacor_lib_QMH_Enqueue Message (poly).vi"("Priority Message? (F)"=TRUE, "Message"="Exit", "Message Queue in"=w325) -> ("error out"=w327:errorcluster)  [unwired: 7 in, 1 out]
              }
              frame True {
                # "If the module was launched externally, calling the Error Reported broadcast VI is the only action performed by the \"Error\" message. The module's caller can then process the error appropriately."
              }
            }
            n135 = Merge Errors(w320, w319) -> (w318:errorcluster)
          }
          frame "Simulate MHL Error" {
            # "#DQMH_HowTo The 'Simulate MHL Error' button  illustrates how the MHL handles errors. This event is instructional in nature and can be removed."
            # "Simulate an error occurring at the MHL"
            n136 = property on="Property Node" class="Mod Admin"(reference=w334) -> ("Accessors:Module ID"=w335:i32)  [unwired: 1 in, 2 out]
            n137 = call "Module Name--constant.vi"("Module ID"=w335) -> ("Module Name"=w330:string)  [unwired: 10 in]
            n138 = Format Into String(format string="Simulated error originating at Message Handling Loop in %s", w330) -> (resulting string=w331:string)  [unwired: 2 in, 1 out]
            n139 = call <vilib>:"Error Cluster From Error Code.vi"("show call chain? (False)"=TRUE, "error message (\"\")"=w331, "error code (0)"=5001) -> ("error out"=w337:errorcluster)  [unwired: 6 in]
            n140 = Merge Errors(w339, w337) -> (w338:errorcluster)
          }
          frame "Exit" {
            w349 = 91  # 91: not all Exit messages will have an argument
            w350 = TRUE  # Stop the VI
            # "Release the message queue reference"
            # "#DQMH_CodeNeeded - Add any required cleanup code here."
            # "Exit - Exit the application."
            n141 = Variant To Data(error in=w357, type=T5 {"Module ID"=-1, "Origin"="", "Exit via Stop Module Req?"=FALSE, "Wait for Module to stop?"=FALSE} ("Stop Argument"), Variant=w348) -> (data=w345:T5, error out=w353:errorcluster)
            n142 = call <vilib>:"Clear Errors.vi"("error in (no error)"=w353, "specific error code to clear (0: all)"=w349) -> ("error out"=w356:errorcluster)  [unwired: 4 in, 1 out]
            n143 = property on="Property Node" class="Mod Admin"(reference=w343) -> ("Accessors:Module ID"=w342:i32)  [unwired: 1 in, 2 out]
            n144 = control-ref of="This VI"() -> (w344:refnum<vi>)
            n145 = call-dynamic "Delacor_lib_QMH_Release Message Queue.vi"("error in"=w356, "Message Queue"=w351) -> ("error out"=w355:errorcluster)  [unwired: 9 in]
            n146 = call "Handle Exit.vi"("Stop Argument"=w345, "Module Admin in"=w343, "VI reference"=w344) -> ("error out"=w354:errorcluster, "Wait for Stop?"=w346:bool)  [unwired: 7 in]
            n147 = Merge Errors(w355, w354) -> (w352:errorcluster)
            n148 = call "Error Reported.vi"("Error"=w352, "Module ID"=w342) -> ()  [unwired: 9 in, 1 out]
            n149 = Unbundle By Name(w341) -> ("VISA resource name"=w340:refnum<visa-resource-name>)
            n150 = call <instrlib>:"Close.vi"("VISA resource name"=w340) -> ()  [unwired: 10 in, 1 out]
          }
          frame Default {
            # "'Default' case only runs if there is a message that isn't defined in any of the other cases.  Output a programming error."
            n151 = property on="Property Node" class="Mod Admin"(reference=w365) -> ("Accessors:Module ID"=w364:i32)  [unwired: 1 in, 2 out]
            n152 = call "Module Name--constant.vi"("Module ID"=w364) -> ("Module Name"=w358:string)  [unwired: 10 in]
            n153 = Format Into String(format string="The invalid message string \"%s\" was received in the Message Handling Loop for module \"%s\".", w359, w358) -> (resulting string=w361:string)  [unwired: 2 in, 1 out]
            n154 = call <vilib>:"Error Cluster From Error Code.vi"("show call chain? (False)"=TRUE, "error message (\"\")"=w361, "error code (0)"=1) -> ("error out"=w367:errorcluster)  [unwired: 6 in]
            n155 = Merge Errors(w368, w367) -> (w369:errorcluster)
          }
        }
        n156 = call-dynamic "Delacor_lib_QMH_Error Handler - Message Handling Loop.vi"("error in"=w223, "Message Queue in"=w214) -> ("dup error in"=w220:errorcluster)  [unwired: 8 in, 1 out]
      }
      n157 = while "DQMH_HELPER_LOOP" {
        shift-right: [w34] -> _
        shift-left: -1 -> [w47]
        shift-right: [w45] -> w23
        shift-left: w22 -> [w46]
        tunnel: w26 -> [w43]
        tunnel: w20 -> [w41]
        shift-right: [w38] -> _
        shift-left: _ -> [w40]
        tunnel: w19 -> [w33]
        stop <- w44 stop-if-true
        w42 = "Continuous Acquisition Tasks HL"  # DQMH_HELPER_LOOP_NAME
        # "Continuous Acquisition Tasks HL"
        n158 = event "DQMH_HELPER_EVENT_STRUCTURE" shown="[1] <CTIWrapper Request Events.Stop Module>: User Event" {
          selector: w46 -> [_ _ _ _]
          dyn-events: [_ _ _ _] -> w45
          timeout: w47 -> [_ _ _ _]
          tunnel: w47 -> [w51 w59 w61 _]
          tunnel: [w51 w59 w62 w73] -> w35
          tunnel: [_ w54 _ _] -> w44
          tunnel: [w49 errorcluster {"status"=FALSE, "code"=0, "source"=""} ("error constant") _ _] -> w37
          tunnel: w43 -> [_ _ _ _]
          tunnel: w41 -> [_ w56 w67 _]
          tunnel: [w52 w55 w63 w74] -> w39
          tunnel: w40 -> [w53 w55 w64 _]
          tunnel: w33 -> [w48 _ _ _]
          event Timeout {
            # "Continous Tasks"
            n159 = event-data() -> ()  [unwired: 1 in, 1 out]
            n160 = call "Read Digital Inptus.vi"("VISA Refnum in"=w53) -> ("error out"=w49:errorcluster, "Digital Inputs"=w50:bool[], "VISA Refnum out"=w52:refnum<visa-resource-name>)  [unwired: 8 in]
            "Digital Inputs" <- w50
            n161 = call "Digital Inptus Updated.vi"("error in"=w49, "Digital Inptus"=w50, "Module ID"=w48) -> ()  [unwired: 8 in, 1 out]
          }
          event User Event {
            n162 = event-data() -> ("Module ID"=w57:i32)  [unwired: 1 in]
            n163 = call "Addressed to This Module.vi"("Module ID from Argument"=w57, "Module Admin"=w56) -> ("Addressed to this instance?"=w54:bool)  [unwired: 8 in, 1 out]
            n164 = case shown="True" w54 {
              tunnel: w55 -> [_ w60]
              frame False {
              }
              frame True {
                n165 = call <instrlib>:"Close.vi"("VISA resource name"=w60) -> ()  [unwired: 10 in, 1 out]
              }
            }
          }
          event User Event {
            n166 = event-data() -> ("Module ID"=w66:i32)  [unwired: 1 in]
            n167 = call "Addressed to This Module.vi"("Module ID from Argument"=w66, "Module Admin"=w67) -> ("Addressed to this instance?"=w65:bool)  [unwired: 8 in, 1 out]
            n168 = case shown="False" w65 {
              tunnel: w64 -> [w69 w72]
              tunnel: [w69 refnum<visa-resource-name> refnum ("VISA resource name")] -> w63
              tunnel: [w68 -1] -> w62
              tunnel: w61 -> [w68 _]
              frame False {
              }
              frame True {
                n169 = call <instrlib>:"Close.vi"("VISA resource name"=w72) -> ()  [unwired: 10 in, 1 out]
              }
            }
          }
          event User Event {
            # "This module called the \"Local Instance.Wake Up CT HL\" local instance request."
            n170 = event-data() -> ("VISA resource name"=w74:refnum<visa-resource-name>)  [unwired: 1 in]
            n171 = call "Continuous Tasks Polling Rate--constant.vi"() -> ("Continuous Tasks Polling Rate"=w73:i32)  [unwired: 11 in]
          }
        }
        n172 = call "Connection Monitor.vi"("Continuous Tasks Polling Rate in"=w35, "error in"=w37, "Module ID"=w33, "VISA Refnum in"=w39) -> ("error out"=w36:errorcluster, "VISA Refnum out"=w38:refnum<visa-resource-name>, "Continuous Tasks Polling Rate out"=w34:i32)  [unwired: 5 in]
        n173 = call-dynamic "Delacor_lib_QMH_Error Handler - Helper Loop.vi"("Error Debug"=w42, "error in"=w36, "Message Queue in"=w43) -> ()  [unwired: 7 in, 2 out]
      }
      n174 = Unregister For Events(event registration refnum=w23) -> ()  [unwired: 1 in, 1 out]
    }
    frame Error {
      n175 = call "Synchronize Caller Events.vi"("Module Admin"=w373) -> ("Module Admin out"=w372:refnum<class "Delacor_lib_QMH_Cloneable Module Admin.lvclass">)  [unwired: 9 in, 1 out]
      n176 = property on="Property Node" class="Mod Admin"(reference=w372) -> ("Accessors:Module ID"=w371:i32)  [unwired: 1 in, 2 out]
      n177 = call-dynamic "Delacor_lib_QMH_Release Message Queue.vi"("error in"=w379, "Message Queue"=w370) -> ("error out"=w378:errorcluster)  [unwired: 9 in]
      n178 = call "Module Name--constant.vi"("Module ID"=w371) -> ("Module Name"=w376:string)  [unwired: 10 in]
      n179 = Format Into String(format string="An error occurred during initialization. %s is no longer running.", w376) -> (resulting string=w374:string)  [unwired: 2 in, 1 out]
      n180 = call "Error Reported.vi"("Additional Information"=w374, "Error"=w378, "Module ID"=w371) -> ()  [unwired: 8 in, 1 out]
    }
  }
  n181 = Merge Errors(w17, w16) -> (w18:errorcluster)
  n182 = call "Close Module.vi"("error in"=w18, "Wait for stop?"=w3, "Module Admin in"=w5) -> ("error out"=w14:errorcluster, "External Launch"=w2:bool, "Module Admin out"=w4:refnum<class "Delacor_lib_QMH_Cloneable Module Admin.lvclass">)  [unwired: 6 in]
  n183 = Unregister For Events(event registration refnum=w9, error in=w14) -> (error out=w13:errorcluster)
  "error out" <- w13
  n184 = case "External Launch?" shown="True" w2 {
    tunnel: w13 -> [_ w380]
    frame False {
    }
    frame True {
      n185 = case shown="No Error" w380 {
        frame No Error {
          n186 = invoke class="VI" method="FP.Close"() -> ()  [unwired: 3 in, 3 out]
        }
        frame Error {
          n187 = disable-structure shown="Default" {
            frame condition #0 (active) {
              n188 = invoke class="VI" method="FP.Open"("Activate"=TRUE ("Activate?")) -> ()  [unwired: 4 in, 5 out]
            }
            frame condition #1 {
              # "Don't show panel on error if running inside a built EXE."
            }
          }
        }
      }
    }
  }
  n189 = local write "Module Admin"(w4) -> ()
